vi "Get Info.vi"(8 "error in (no error)":errorcluster, 11 "ACreditAccount in":refnum<class "ACreditAccount.lvclass">) -> (0 "error out":errorcluster, 2 "Account Information":T1, 3 "ACreditAccount out":refnum<class "ACreditAccount.lvclass">)   [LabVIEW 2020, in "ACreditAccount.lvclass"]
uses:
  ACreditAccount.lvclass
  Account Information STYP.ctl
  ACreditAccount.lvclass/ACreditAccount.ctl
  AInterestAccount/AInterestAccount.lvclass
  IInfoable/IInfoable.lvclass
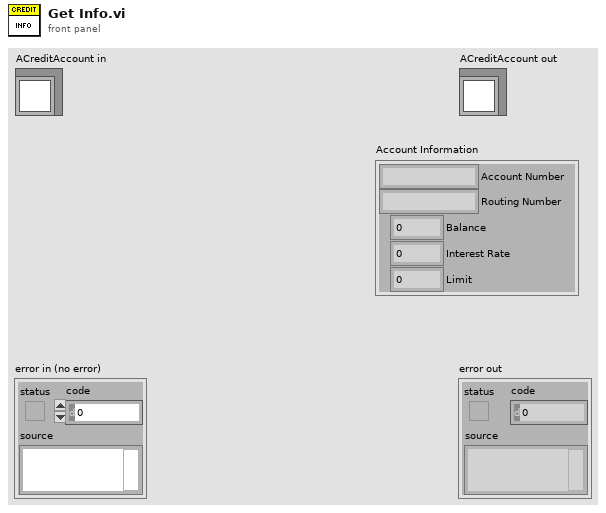
[diagram p1: front panel]
types:
  T1 = typedef "IInfoable.lvclass/Account Information STYP.ctl" = cluster{"Account Number":string, "Routing Number":string, "Balance":dbl, "Interest Rate":dbl, "Limit":dbl}
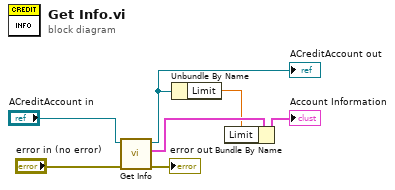
[diagram p0: block diagram]
diagram:
  n1 = call-parent "Get Info.vi"("error in (no error)"="error in (no error)", "AInterestAccount in"="ACreditAccount in") -> ("error out"=→"error out":errorcluster, "Account Information"=w6:T1, "AInterestAccount out"=w2:refnum<class "ACreditAccount.lvclass">)  [unwired: 7 in]
  "ACreditAccount out" <- w2
  n2 = Unbundle By Name(w2) -> ("Limit"=w1:dbl)
  n3 = Bundle By Name(cluster=w6, "Limit"=w1) -> (→"Account Information":T1)
